vi "BIO New Connect Client Test.vi"() -> ()   [LabVIEW 2013]
uses:
  SSL_Lib/SSL-Lib/SSL-Lib.lvclass
  SSL_Lib/SSL-Context/SSL-Context.lvclass
  SSL_Lib/BIO/BIO.lvclass
  SSL_Lib/SSL/SSL.lvclass
  SSL_Lib/SSL/SSL_Mode.ctl
  SSL_Lib/SSL-Lib/Library Paths.ctl
  SSL_Lib/SSL-Context/SSL Options.ctl
  SSL_Lib/SSL-Context/SSL Verify Mode.ctl
  SSL_Lib/X509-Cert/X509-Cert.lvclass
  SSL_Lib/SSL/X509_Host_Verify_Flags.ctl
  SSL_Lib/SSL/X509_Verify_Result.ctl
panel:
  out "verify result":T1
  out "issuer name":string
  out "subject name":string
  out "String read":string
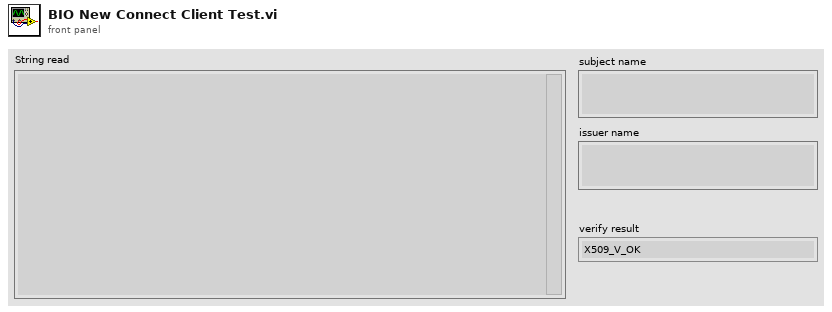
[diagram p1: front panel]
types:
  T1 = typedef "SSL_Lib.lvlib/SSL.lvclass/X509_Verify_Result.ctl" = enum16{"X509_V_OK", "X509_V_ERR_UNSPECIFIED", "X509_V_ERR_UNABLE_TO_GET_ISSUER_CERT", "X509_V_ERR_UNABLE_TO_GET_CRL", "X509_V_ERR_UNABLE_TO_DECRYPT_CERT_SIGNATURE", "X509_V_ERR_UNABLE_TO_DECRYPT_CRL_SIGNATURE", "X509_V_ERR_UNABLE_TO_DECODE_ISSUER_PUBLIC_KEY", "X509_V_ERR_CERT_SIGNATURE_FAILURE", "X509_V_ERR_CRL_SIGNATURE_FAILURE", "X509_V_ERR_CERT_NOT_YET_VALID", "X509_V_ERR_CERT_HAS_EXPIRED", "X509_V_ERR_CRL_NOT_YET_VALID", "X509_V_ERR_CRL_HAS_EXPIRED", "X509_V_ERR_ERROR_IN_CERT_NOT_BEFORE_FIELD", "X509_V_ERR_ERROR_IN_CERT_NOT_AFTER_FIELD", "X509_V_ERR_ERROR_IN_CRL_LAST_UPDATE_FIELD", "X509_V_ERR_ERROR_IN_CRL_NEXT_UPDATE_FIELD", "X509_V_ERR_OUT_OF_MEM", "X509_V_ERR_DEPTH_ZERO_SELF_SIGNED_CERT", "X509_V_ERR_SELF_SIGNED_CERT_IN_CHAIN", "X509_V_ERR_UNABLE_TO_GET_ISSUER_CERT_LOCALLY", "X509_V_ERR_UNABLE_TO_VERIFY_LEAF_SIGNATURE", "X509_V_ERR_CERT_CHAIN_TOO_LONG", "X509_V_ERR_CERT_REVOKED", "X509_V_ERR_INVALID_CA", "X509_V_ERR_PATH_LENGTH_EXCEEDED", "X509_V_ERR_INVALID_PURPOSE", "X509_V_ERR_CERT_UNTRUSTED", "X509_V_ERR_CERT_REJECTED", "X509_V_ERR_SUBJECT_ISSUER_MISMATCH", "X509_V_ERR_AKID_SKID_MISMATCH", "X509_V_ERR_AKID_ISSUER_SERIAL_MISMATCH", "X509_V_ERR_KEYUSAGE_NO_CERTSIGN", "X509_V_ERR_UNABLE_TO_GET_CRL_ISSUER", "X509_V_ERR_UNHANDLED_CRITICAL_EXTENSION", "X509_V_ERR_KEYUSAGE_NO_CRL_SIGN", "X509_V_ERR_UNHANDLED_CRITICAL_CRL_EXTENSION", "X509_V_ERR_INVALID_NON_CA", "X509_V_ERR_PROXY_PATH_LENGTH_EXCEEDED", "X509_V_ERR_KEYUSAGE_NO_DIGITAL_SIGNATURE", "X509_V_ERR_PROXY_CERTIFICATES_NOT_ALLOWED", "X509_V_ERR_INVALID_EXTENSION", "X509_V_ERR_INVALID_POLICY_EXTENSION", "X509_V_ERR_NO_EXPLICIT_POLICY", "X509_V_ERR_DIFFERENT_CRL_SCOPE", "X509_V_ERR_UNSUPPORTED_EXTENSION_FEATURE", "X509_V_ERR_UNNESTED_RESOURCE", "X509_V_ERR_PERMITTED_VIOLATION", "X509_V_ERR_EXCLUDED_VIOLATION", "X509_V_ERR_SUBTREE_MINMAX", "X509_V_ERR_APPLICATION_VERIFICATION", "X509_V_ERR_UNSUPPORTED_CONSTRAINT_TYPE", "X509_V_ERR_UNSUPPORTED_CONSTRAINT_SYNTAX", "X509_V_ERR_UNSUPPORTED_NAME_SYNTAX", "X509_V_ERR_CRL_PATH_VALIDATION_ERROR", "N/A", "X509_V_ERR_SUITE_B_INVALID_VERSION", "X509_V_ERR_SUITE_B_INVALID_ALGORITHM", "X509_V_ERR_SUITE_B_INVALID_CURVE", "X509_V_ERR_SUITE_B_INVALID_SIGNATURE_ALGORITHM", "X509_V_ERR_SUITE_B_LOS_NOT_ALLOWED", "X509_V_ERR_SUITE_B_CANNOT_SIGN_P_384_WITH_P_256", "X509_V_ERR_HOSTNAME_MISMATCH", "X509_V_ERR_EMAIL_MISMATCH", "X509_V_ERR_IP_ADDRESS_MISMATCH", "X509_V_ERR_INVALID_CALL", "X509_V_ERR_STORE_LOOKUP", "X509_V_ERR_PROXY_SUBJECT_NAME_VIOLATION"}
  T2 = typedef "SSL_Lib.lvlib/SSL.lvclass/SSL_Mode.ctl" = i32
  T3 = typedef "SSL_Lib.lvlib/SSL-Context.lvclass/SSL Options.ctl" = i32
  T4 = typedef "SSL_Lib.lvlib/SSL-Lib.lvclass/Library Paths.ctl" = cluster{"SSL Library Path":path, "Crypto Library Path":path}
  T5 = typedef "SSL_Lib.lvlib/SSL-Context.lvclass/SSL Verify Mode.ctl" = i32
  T6 = typedef "SSL_Lib.lvlib/SSL.lvclass/X509_Host_Verify_Flags.ctl" = u32
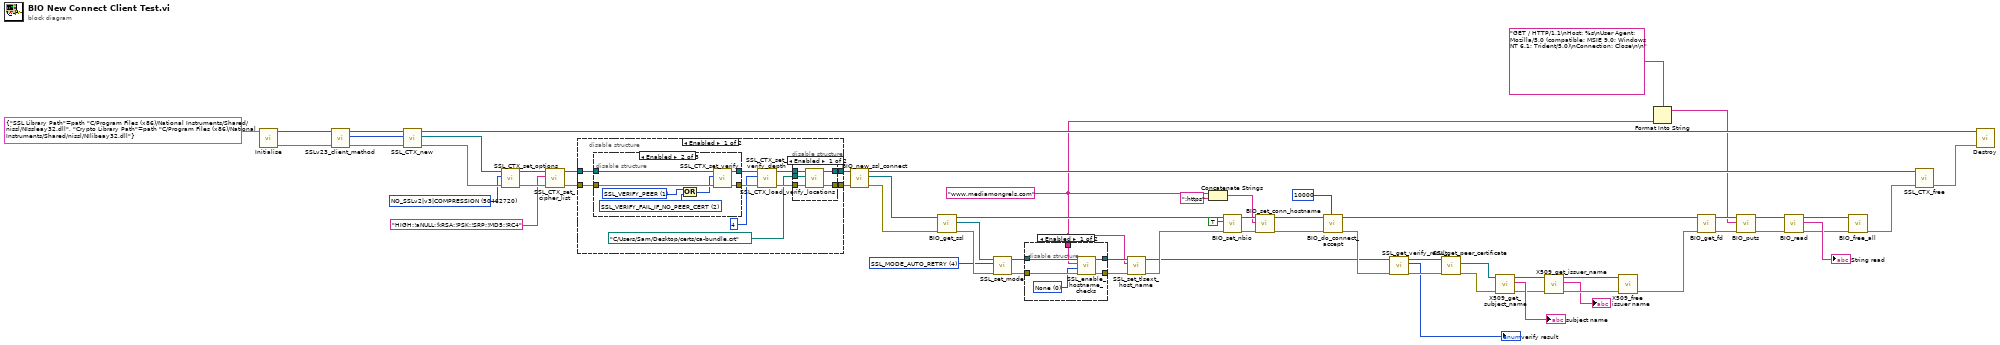
[diagram p0: block diagram]
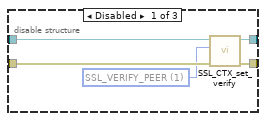
[diagram p3: hidden frame]
diagram:
  w1 = "www.mediamongrels.com" ("Hostname")
  w32 = T2 4 items=["None"=0, "SSL_MODE_ENABLE_PARTIAL_WRITE"=1, "SSL_MODE_ACCEPT_MOVING_WRITE_BUFFER"=2, "SSL_MODE_AUTO_RETRY"=4, "SSL_MODE_RELEASE_BUFFERS"=16, "SSL_MODE_SEND_FALLBACK_SCSV"=128] ("Mode")
  w33 = T3 50462720 items=["None"=0, "NO_SSLv2|v3|COMPRESSION"=50462720, "SSL_OP_NO_COMPRESSION"=131072, "SSL_OP_NO_SSLv2"=16777216, "SSL_OP_NO_SSLv3"=33554432, "SSL_OP_NO_TLSv1"=67108864, "SSL_OP_NO_TLSv1_2"=134217728, "SSL_OP_NO_TLSv1_1"=268435456] ("Options")
  n1 = call "Initialise.vi"("Library Paths"=T4 {"SSL Library Path"=path "C:/Program Files (x86)/National Instruments/Shared/nissl/NIssleay32.dll", "Crypto Library Path"=path "C:/Program Files (x86)/National Instruments/Shared/nissl/NIlibeay32.dll"}) -> ("error out"=w60:errorcluster, "SSL-Lib out"=w64:refnum<class "SSL-Lib.lvclass">)  [unwired: 9 in]
  n2 = call "SSLv23_client_method.vi"("error in (no error)"=w60, "SSL-Lib in"=w64) -> ("error out"=w58:errorcluster, "*SSL_Method"=w63:u64, "SSL-Lib out"=w62:refnum<class "SSL-Lib.lvclass">)  [unwired: 7 in]
  n3 = call "SSL_CTX_new.vi"("error in (no error)"=w58, "*SSL_Method"=w63, "SSL-Lib in"=w62) -> ("error out"=w34:errorcluster, "SSL-Context out"=w35:refnum<class "SSL-Context.lvclass">, "SSL-Lib out"=w57:refnum<class "SSL-Lib.lvclass">)  [unwired: 6 in]
  n4 = call "SSL_CTX_set_options.vi"("error in (no error)"=w34, "Options"=w33, "SSL-Context in"=w35) -> ("error out"=w13:errorcluster, "SSL-Context out"=w16:refnum<class "SSL-Context.lvclass">)  [unwired: 7 in]
  n5 = call "SSL_CTX_set_cipher_list.vi"("error in (no error)"=w13, "Cipher List"="HIGH:!aNULL:!kRSA:!PSK:!SRP:!MD5:!RC4", "SSL-Context in"=w16) -> ("error out"=w14:errorcluster, "SSL-Context out"=w15:refnum<class "SSL-Context.lvclass">)  [unwired: 7 in]
  n6 = disable-structure shown="Enabled" {
    disable-tunnel: [w74 w97] -> w31
    disable-tunnel: [w73 w96] -> w30
    disable-tunnel: w15 -> [w72 w97]
    disable-tunnel: w14 -> [w71 w96]
    frame Enabled {
      n7 = disable-structure shown="Enabled" {
        disable-tunnel: w72 -> [w79 w86 w88]
        disable-tunnel: w71 -> [w78 w85 w87]
        disable-tunnel: [w77 w84 w87] -> w70
        disable-tunnel: [w76 w83 w88] -> w69
        frame Disabled {
          w75 = T5 1 items=["SSL_VERIFY_NONE"=0, "SSL_VERIFY_PEER"=1, "SSL_VERIFY_FAIL_IF_NO_PEER_CERT"=2, "SSL_VERIFY_CLIENT_ONCE"=4] ("Mode")
          n8 = call "SSL_CTX_set_verify.vi"("error in (no error)"=w78, "Mode"=w75, "SSL-Context in"=w79) -> ("error out"=w77:errorcluster, "SSL-Context out"=w76:refnum<class "SSL-Context.lvclass">)  [unwired: 7 in]
        }
        frame Enabled {
          w82 = T5 2 items=["SSL_VERIFY_NONE"=0, "SSL_VERIFY_PEER"=1, "SSL_VERIFY_FAIL_IF_NO_PEER_CERT"=2, "SSL_VERIFY_CLIENT_ONCE"=4] ("Mode")
          w81 = T5 1 items=["SSL_VERIFY_NONE"=0, "SSL_VERIFY_PEER"=1, "SSL_VERIFY_FAIL_IF_NO_PEER_CERT"=2, "SSL_VERIFY_CLIENT_ONCE"=4] ("Mode")
          n9 = Or(x=w81, y=w82) -> (x .or. y?=w80:T5)
          n10 = call "SSL_CTX_set_verify.vi"("error in (no error)"=w85, "Mode"=w80, "SSL-Context in"=w86) -> ("error out"=w84:errorcluster, "SSL-Context out"=w83:refnum<class "SSL-Context.lvclass">)  [unwired: 7 in]
        }
        frame Disabled {
        }
      }
      n11 = call "SSL_CTX_set_verify_depth.vi"("error in (no error)"=w70, "Depth"=4, "SSL-Context in"=w69) -> ("error out"=w66:errorcluster, "SSL-Context out"=w67:refnum<class "SSL-Context.lvclass">)  [unwired: 7 in]
      n12 = disable-structure shown="Enabled" {
        disable-tunnel: [w93 w95] -> w74
        disable-tunnel: [w92 w94] -> w73
        disable-tunnel: w67 -> [w91 w95]
        disable-tunnel: w66 -> [w90 w94]
        disable-tunnel: path "C:/Users/Sam/Desktop/certs/ca-bundle.crt" ("Path to CA bundle") -> [w89 _]
        frame Enabled {
          n13 = call "SSL_CTX_load_verify_locations.vi"("error in (no error)"=w90, "Path to CA bundle"=w89, "SSL-Context in"=w91) -> ("error out"=w92:errorcluster, "SSL-Context out"=w93:refnum<class "SSL-Context.lvclass">)  [unwired: 7 in]
        }
        frame Disabled {
        }
      }
    }
    frame Disabled {
    }
  }
  n14 = call "BIO_new_ssl_connect.vi"("error in (no error)"=w30, "SSL-Context in"=w31) -> ("error out"=w53:errorcluster, "BIO out"=w54:refnum<class "BIO.lvclass">, "SSL-Context out"=w56:refnum<class "SSL-Context.lvclass">)  [unwired: 7 in]
  n15 = call "BIO_get_ssl.vi"("error in (no error)"=w53, "BIO in"=w54) -> ("error out"=w51:errorcluster, "SSL out"=w52:refnum<class "SSL.lvclass">, "BIO out"=w44:refnum<class "BIO.lvclass">)  [unwired: 7 in]
  n16 = call "SSL_set_mode.vi"("error in (no error)"=w51, "Mode"=w32, "SSL in"=w52) -> ("error out"=w11:errorcluster, "SSL out"=w10:refnum<class "SSL.lvclass">)  [unwired: 7 in]
  n17 = disable-structure shown="Enabled" {
    disable-tunnel: w11 -> [w103 w104]
    disable-tunnel: w10 -> [w102 w105]
    disable-tunnel: [w101 w104] -> w4
    disable-tunnel: [w100 w105] -> w5
    disable-tunnel: w1 -> [w98 _]
    frame Enabled {
      w99 = T6 0 items=["None"=0, "X509_CHECK_FLAG_ALWAYS_CHECK_SUBJECT"=1, "X509_CHECK_FLAG_NO_WILDCARDS"=2, "X509_CHECK_FLAG_NO_PARTIAL_WILDCARDS"=4, "X509_CHECK_FLAG_MULTI_LABEL_WILDCARDS"=8, "X509_CHECK_FLAG_SINGLE_LABEL_SUBDOMAINS"=16] ("Verification Flags")
      n18 = call "SSL_enable_hostname_checks.vi"("error in (no error)"=w103, "Verification Flags"=w99, "Hostname"=w98, "SSL in"=w102) -> ("error out"=w101:errorcluster, "SSL out"=w100:refnum<class "SSL.lvclass">)  [unwired: 6 in]
    }
    frame Disabled {
    }
  }
  n19 = call "SSL_set_tlsext_host_name.vi"("error in (no error)"=w4, "Hostname"=w1, "SSL in"=w5) -> ("error out"=w3:errorcluster, "SSL out"=w2:refnum<class "SSL.lvclass">)  [unwired: 7 in]
  n20 = Concatenate Strings(w1, ":https" ("string")) -> (w8:string)
  n21 = call "BIO_set_nbio.vi"("error in (no error)"=w3, "Non-Blocking?"=TRUE, "BIO in"=w44) -> ("error out"=w45:errorcluster, "BIO out"=w42:refnum<class "BIO.lvclass">)  [unwired: 7 in]
  n22 = call "BIO_set_conn_hostname.vi"("error in (no error)"=w45, "Hostname"=w8, "BIO in"=w42) -> ("error out"=w40:errorcluster, "BIO out"=w41:refnum<class "BIO.lvclass">)  [unwired: 7 in]
  n23 = call "BIO_do_connect_accept.vi"("Timeout (10000ms)"=u32 10000, "error in (no error)"=w40, "BIO in"=w41) -> ("error out"=w20:errorcluster, "BIO out"=w39:refnum<class "BIO.lvclass">)  [unwired: 7 in]
  n24 = call "SSL_get_verify_result.vi"("error in (no error)"=w20, "SSL-Lib in"=w2) -> ("error out"=w19:errorcluster, "verify result"=→"verify result":T1, "SSL-Lib out"=w18:refnum<class "SSL.lvclass">)  [unwired: 7 in]
  n25 = call "SSL_get_peer_certificate.vi"("error in (no error)"=w19, "SSL-Lib in"=w18) -> ("error out"=w27:errorcluster, "X509-Cert out"=w28:refnum<class "X509-Cert.lvclass">)  [unwired: 7 in, 1 out]
  n26 = call "X509_get_subject_name.vi"("error in (no error)"=w27, "X509-Cert in"=w28) -> ("error out"=w23:errorcluster, "subject name"=→"subject name":string, "X509-Cert out"=w25:refnum<class "X509-Cert.lvclass">)  [unwired: 7 in]
  n27 = call "X509_get_issuer_name.vi"("error in (no error)"=w23, "X509-Cert in"=w25) -> ("error out"=w22:errorcluster, "issuer name"=→"issuer name":string, "X509-Cert out"=w24:refnum<class "X509-Cert.lvclass">)  [unwired: 7 in]
  n28 = call "X509_free.vi"("error in (no error)"=w22, "X509-Cert in"=w24) -> ("error out"=w29:errorcluster)  [unwired: 9 in]
  n29 = Format Into String(format string="GET / HTTP/1.1\nHost: %s\nUser Agent: Mozilla/5.0 (compatible; MSIE 9.0; Windows NT 6.1; Trident/5.0)\nConnection: Close\n\n" ("String to write"), w1) -> (resulting string=w6:string)  [unwired: 2 in, 1 out]
  n30 = call "BIO_get_fd.vi"("error in (no error)"=w29, "BIO in"=w39) -> ("error out"=w38:errorcluster, "BIO out"=w37:refnum<class "BIO.lvclass">)  [unwired: 7 in, 1 out]
  n31 = call "BIO_puts.vi"("error in (no error)"=w38, "String to write"=w6, "BIO in"=w37) -> ("error out"=w50:errorcluster, "BIO out"=w49:refnum<class "BIO.lvclass">)  [unwired: 7 in]
  n32 = call "BIO_read.vi"("error in (no error)"=w50, "BIO in"=w49) -> ("error out"=w46:errorcluster, "String read"=→"String read":string, "BIO out"=w48:refnum<class "BIO.lvclass">)  [unwired: 7 in]
  n33 = call "BIO_free_all.vi"("error in (no error)"=w46, "BIO in"=w48) -> ("error out"=w55:errorcluster)  [unwired: 9 in]
  n34 = call "SSL_CTX_free.vi"("error in (no error)"=w55, "SSL-Context in"=w56) -> ("error out"=w59:errorcluster)  [unwired: 9 in]
  n35 = call "Destroy.vi"("error in (no error)"=w59, "SSL-Lib in"=w57) -> ()  [unwired: 9 in, 1 out]
